vi "AH Average Time Setupvi.vi"(10 "Averaging Time Labels":string[](array[string]), 11 "Current Setting":u32) -> (2 "Avg Time (mS)":u32, 3 "Min Avg":dbl)   [LabVIEW 2020]
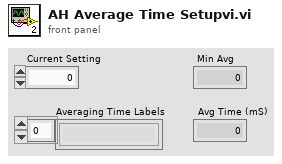
[diagram p1: front panel]
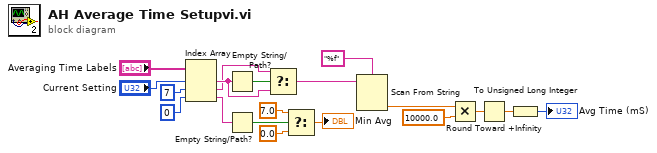
[diagram p0: block diagram]
diagram:
  n1 = Index Array(array="Averaging Time Labels", index #1="Current Setting", index #2=7 ("index"), index #3=0 ("index")) -> (element #1=w18:string, element #2=w17:string, element #3=w15:string)
  n2 = Empty String/Path?(string/path=w18) -> (empty?=w16:bool)
  n3 = Empty String/Path?(string/path=w15) -> (empty?=w9:bool)
  n4 = Select(t=w17, s=w16, f=w18) -> (s? t:f=w19:string)
  n5 = Select(t=7.0, s=w9, f=0.0) -> (s? t:f=→"Min Avg":dbl)
  n6 = Scan From String(format string="%f", input string=w19) -> (output 1=w4:dbl)  [unwired: 3 in, 3 out]
  n7 = Multiply(x=w4, y=10000.0 ("x")) -> (x*y=w3:dbl)
  n8 = Round Toward +Infinity(x=w3) -> (ceil(x): smallest int >= x=w1:dbl)
  n9 = To Unsigned Long Integer(number=w1) -> (unsigned 32bit integer=→"Avg Time (mS)":u32)
